vi "4461 - Create IO Channels Parallel Uneven.vi"(0 "sample mode":i32(ring)=10178 items=["Finite Samples"=10178, "Continuous Samples"=10123], 1 "Channels: Lockin":T1={"REF f (Hz)"=[0.4, 0.4], "REF phi (deg)"=[0.0, 0.0]} {"REF phi (deg)" format="%#_3g"}, 6 "error in":errorcluster, 7 "AI Buffer Size (S)":i32=10, 8 "sampling info":cluster{"Fs":dbl, "#s":dbl}, 9 "AO":T2={"AO amp (V)"=[0.1, 0.09, 0.08, 0.07, 0.06, 0.05, 0.04, 0.03], "AO DC (V)"=[0.0, 0.0, 0.0, 0.0, 0.0, 0.0, 0.0, 0.0], "AO f (Hz)"=[13.0, 13.0, 13.0, 13.0, 13.0, 13.0, 13.0, 13.0], "AO phi (deg)"=[0.0, 0.0, 0.0, 0.0, 0.0, 0.0, 0.0, 0.0], "function"=[enum."Sine Wave", enum."Sine Wave", enum."Sine Wave", enum."Sine Wave", enum."Sine Wave", enum."Sine Wave", enum."Sine Wave", enum."Sine Wave"]} {"AO DC (V)" format="%#_6p"; "AO amp (V)" format="%#_6p"}, 10 "AO Configuration":T3(array[cluster]), 11 "AI Configuration":T4(array[cluster])) -> (2 "AO Task":refnum<k21>[](array[refnum]), 3 "AI task":refnum<k21>[](array[refnum]), 4 "error out":errorcluster, 5 "phase log":dbl[](array[numeric])=[0.99999999999938, 0.99999999999938])   [LabVIEW 2016]
uses:
  <vilib>/DAQmx/write.llb/DAQmx Write (Analog 1D Wfm NChan NSamp).vi
  <vilib>/DAQmx/read.llb/DAQmx Read (Analog 1D Wfm NChan NSamp).vi
  <vilib>/DAQmx/create/channels.llb/DAQmx Create Channel (AI-Voltage-Basic).vi
  <vilib>/DAQmx/configure/timing.llb/DAQmx Timing (Sample Clock).vi
  <vilib>/DAQmx/create/channels.llb/DAQmx Create Channel (AO-Voltage-Basic).vi
  <vilib>/DAQmx/configure/trigger.llb/DAQmx Start Trigger (Digital Edge).vi
  <vilib>/DAQmx/miscellaneous.llb/DAQmx Fill In Error Info.vi
  <resource>/objmgr/daqmx.rc
panel:
  in  "AI.FilterDelay":dbl
  in  "AI.Gain":dbl
  in  "input terminal configuration":i32(ring)=-1 items=["default"=-1, "RSE"=10083, "NRSE"=10078, "Differential"=10106, "Pseudodifferential"=12529]
  in  "output terminal configuration":i32(ring)=-1 items=["Default"=-1, "RSE"=10083, "Differential"=10106, "Pseudodifferential"=12529]
  in  "SampClk.Timebase.Rate":dbl
  in  "SampQuant.SampPerChan":dbl
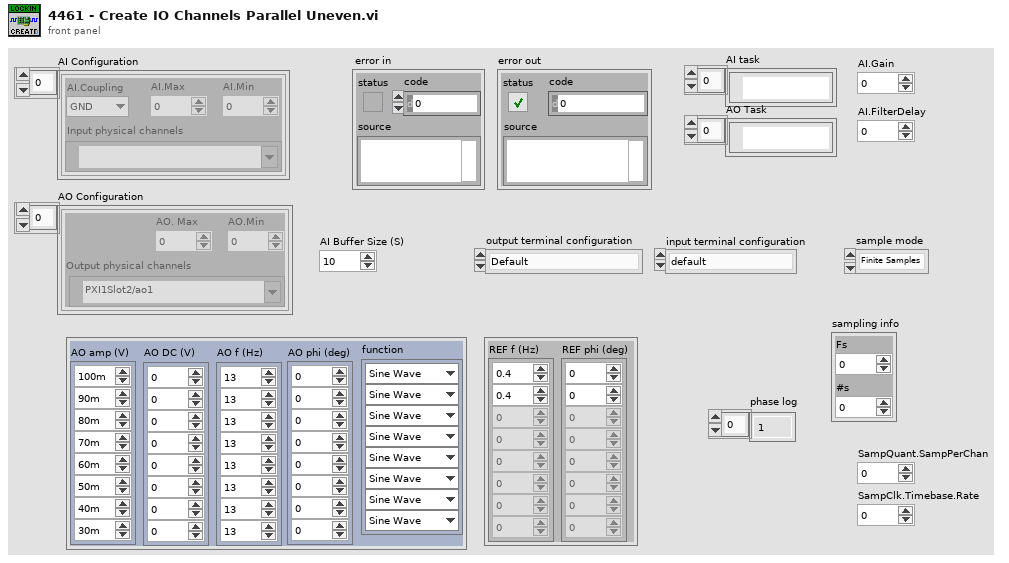
[diagram p1: front panel]
types:
  T1 = cluster{"REF f (Hz)":dbl[], "REF phi (deg)":dbl[]}
  T2 = cluster{"AO amp (V)":dbl[], "AO DC (V)":dbl[], "AO f (Hz)":dbl[], "AO phi (deg)":dbl[], "function":enum16{"Sine Wave", "Triangle Wave", "Square Wave", "Sawtooth Wave"}[]}
  T3 = cluster{"Output physical channels":tag, "AO. Max":dbl, "AO.Min":dbl}[]
  T4 = cluster{"AI.Coupling":enum16{"AC", "DC", "GND"}, "AI.Max":dbl, "AI.Min":dbl, "Input physical channels":tag}[]
  T5 = cluster{"Output physical channels":tag, "AO. Max":dbl, "AO.Min":dbl}
  T6 = cluster{"AI.Coupling":enum16{"AC", "DC", "GND"}, "AI.Max":dbl, "AI.Min":dbl, "Input physical channels":tag}
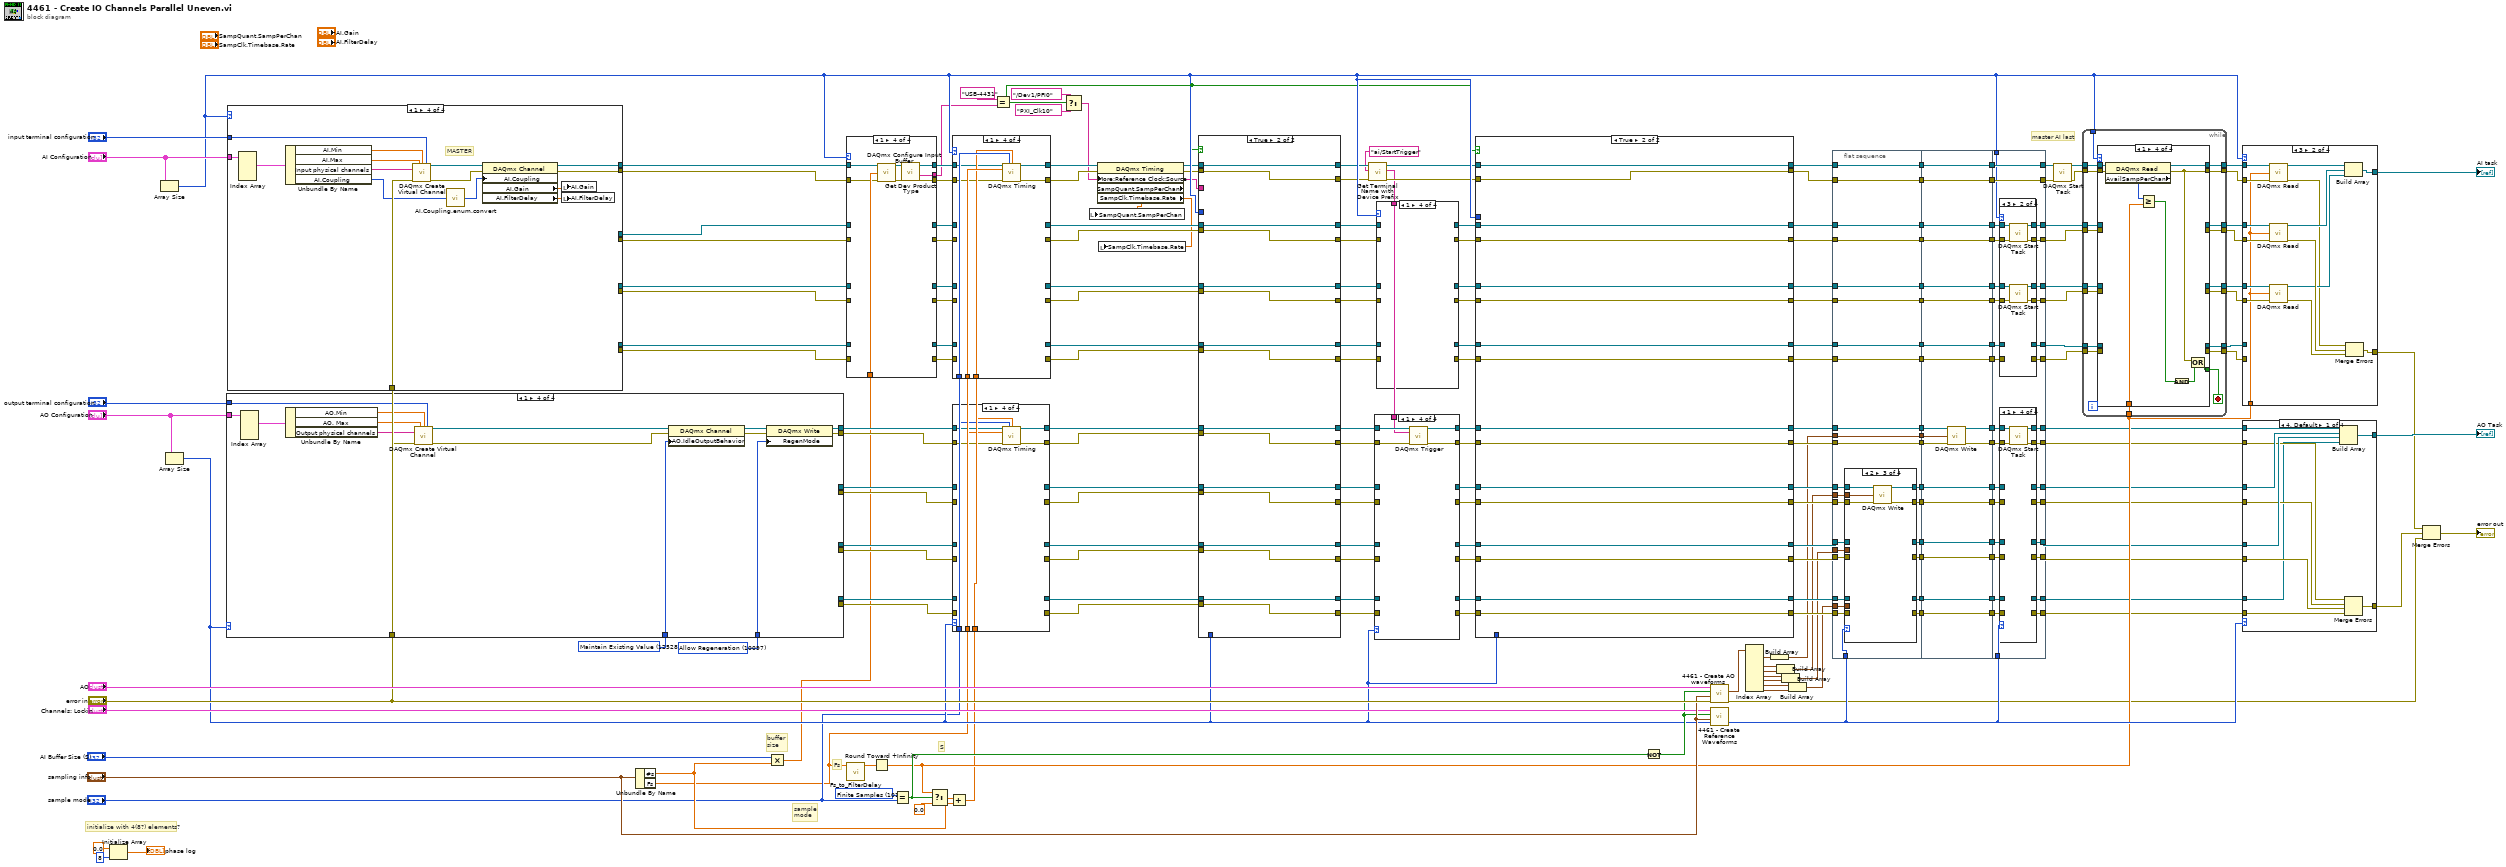
[diagram p0: block diagram]
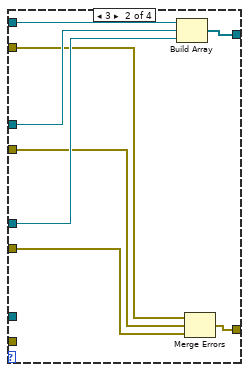
[diagram p2: hidden frame]
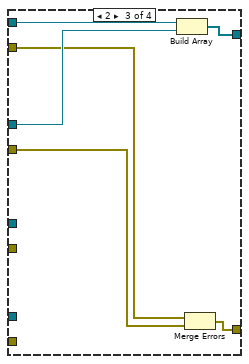
[diagram p3: hidden frame]
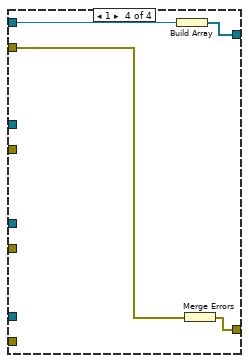
[diagram p4: hidden frame]
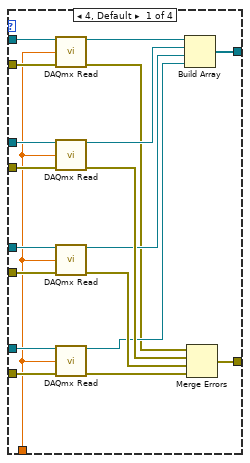
[diagram p5: hidden frame]
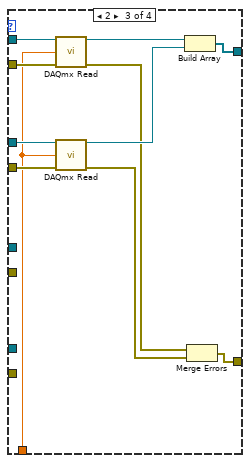
[diagram p6: hidden frame]
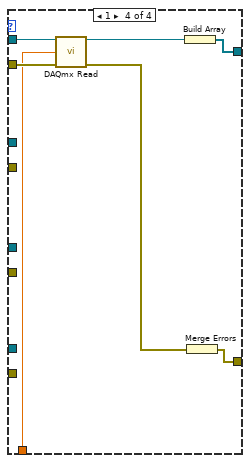
[diagram p7: hidden frame]
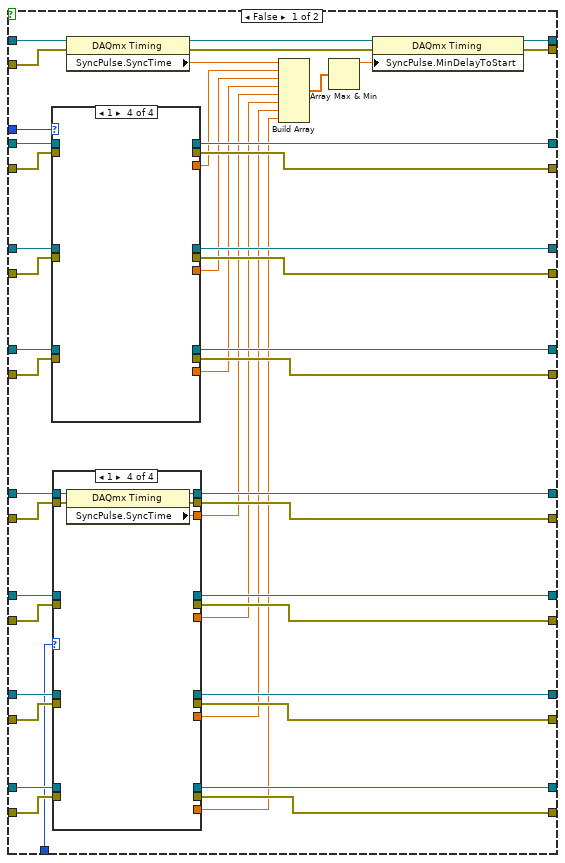
[diagram p8: hidden frame]
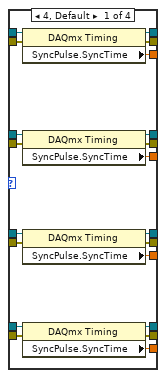
[diagram p9: hidden frame]
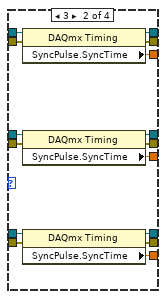
[diagram p10: hidden frame]
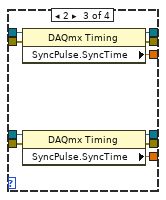
[diagram p11: hidden frame]
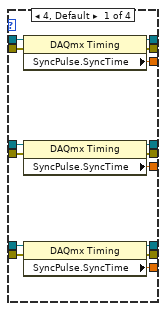
[diagram p12: hidden frame]
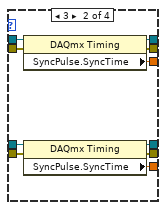
[diagram p13: hidden frame]
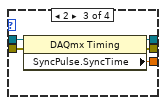
[diagram p14: hidden frame]
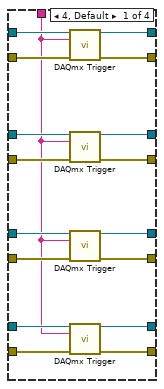
[diagram p15: hidden frame]
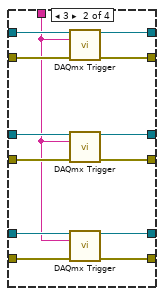
[diagram p16: hidden frame]
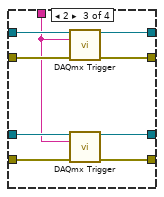
[diagram p17: hidden frame]
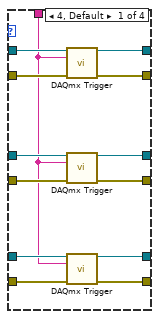
[diagram p18: hidden frame]
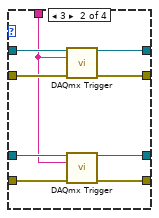
[diagram p19: hidden frame]
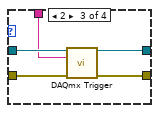
[diagram p20: hidden frame]
diagram:
  w186 = 10097 items=["Allow Regeneration"=10097, "Do Not Allow Regeneration"=10158] ("RegenMode")
  w188 = 12528 items=["Zero Volts"=12526, "High-Impedance"=12527, "Maintain Existing Value"=12528] ("AO.IdleOutputBehavior")
  w191 = 10178 items=["Finite Samples"=10178, "Continuous Samples"=10123] ("sample mode 2")
  # "master AI last"
  # "S"
  # "Fs"
  # "sample\nmode"
  # "buffer\nsize"
  # "initialize with 4(8?) elements?"
  n1 = Initialize Array(0.0 ("element"), 8 ("dimension size")) -> (→"phase log":dbl[])
  n2 = Array Size(array="AI Configuration") -> (size(s)=w179:i32)
  n3 = Array Size(array="AO Configuration") -> (size(s)=w181:i32)
  n4 = case shown="1" w181 {
    tunnel: "AO Configuration" -> [w250 w285 w310 w325]
    tunnel: "error in" -> [w242 w278 w304 w320]
    tunnel: "output terminal configuration" -> [w241 w277 w303 w319]
    tunnel: [w236 w272 w298 w314] -> w79
    tunnel: [w235 _ _ _] -> w78
    tunnel: [w234 w271 w297 _] -> w77
    tunnel: [w233 w270 _ _] -> w76
    tunnel: w188 -> [w232 w269 w296 w313]
    tunnel: [w231 w268 w295 w312] -> w58
    tunnel: [w230 w267 w294 _] -> w57
    tunnel: [w229 w266 _ _] -> w56
    tunnel: [w228 _ _ _] -> w55
    tunnel: w186 -> [w227 w265 w293 w311]
    frame 4, Default {
      n5 = Index Array(array=w250) -> (element #1=w249:T5, element #2=w243:T5, element #3=w244:T5, element #4=w245:T5)  [unwired: 4 in]
      n6 = Unbundle By Name(w249) -> ("AO.Min"=w246:dbl, "AO. Max"=w247:dbl, "Output physical channels"=w248:tag)
      n7 = Unbundle By Name(w243) -> ("AO.Min"=w226:dbl, "AO. Max"=w225:dbl, "Output physical channels"=w224:tag)
      n8 = Unbundle By Name(w244) -> ("AO.Min"=w221:dbl, "AO. Max"=w222:dbl, "Output physical channels"=w223:tag)
      n9 = Unbundle By Name(w245) -> ("AO.Min"=w220:dbl, "AO. Max"=w219:dbl, "Output physical channels"=w218:tag)
      n10 = call-poly <vilib>:"DAQmx Create Virtual Channel.vi"("maximum value"=w247, "minimum value"=w246, "output terminal configuration"=w241, "physical channels"=w248, "error in"=w242) -> ("task out"=w240:refnum<k21>, "error out"=w239:errorcluster)  [unwired: 9 in]
      n11 = call-poly <vilib>:"DAQmx Create Virtual Channel.vi"("maximum value"=w225, "minimum value"=w226, "output terminal configuration"=w241, "physical channels"=w224, "error in"=w242) -> ("task out"=w212:refnum<k21>, "error out"=w213:errorcluster)  [unwired: 9 in]
      n12 = call-poly <vilib>:"DAQmx Create Virtual Channel.vi"("maximum value"=w222, "minimum value"=w221, "output terminal configuration"=w241, "physical channels"=w223, "error in"=w242) -> ("task out"=w214:refnum<k21>, "error out"=w215:errorcluster)  [unwired: 9 in]
      n13 = call-poly <vilib>:"DAQmx Create Virtual Channel.vi"("maximum value"=w219, "minimum value"=w220, "output terminal configuration"=w241, "physical channels"=w218, "error in"=w242) -> ("task out"=w217:refnum<k21>, "error out"=w216:errorcluster)  [unwired: 9 in]
      n14 = property class="DAQmx Channel"(reference=w240, error in=w239, "AO.IdleOutputBehavior"=w232) -> (reference out=w238:refnum<k21>, error out=w237:errorcluster)
      n15 = property class="DAQmx Channel"(reference=w212, error in=w213, "AO.IdleOutputBehavior"=w232) -> (reference out=w206:refnum<k21>, error out=w207:errorcluster)
      n16 = property class="DAQmx Channel"(reference=w214, error in=w215, "AO.IdleOutputBehavior"=w232) -> (reference out=w208:refnum<k21>, error out=w209:errorcluster)
      n17 = property class="DAQmx Channel"(reference=w217, error in=w216, "AO.IdleOutputBehavior"=w232) -> (reference out=w211:refnum<k21>, error out=w210:errorcluster)
      n18 = property class="DAQmx Write"(reference=w238, error in=w237, "RegenMode"=w227) -> (reference out=w236:refnum<k21>, error out=w231:errorcluster)
      n19 = property class="DAQmx Write"(reference=w206, error in=w207, "RegenMode"=w227) -> (reference out=w234:refnum<k21>, error out=w230:errorcluster)
      n20 = property class="DAQmx Write"(reference=w208, error in=w209, "RegenMode"=w227) -> (reference out=w233:refnum<k21>, error out=w229:errorcluster)
      n21 = property class="DAQmx Write"(reference=w211, error in=w210, "RegenMode"=w227) -> (reference out=w235:refnum<k21>, error out=w228:errorcluster)
    }
    frame 3 {
      n22 = Index Array(array=w285) -> (element #1=w284:T5, element #2=w279:T5, element #3=w280:T5)  [unwired: 4 in, 1 out]
      n23 = Unbundle By Name(w284) -> ("AO.Min"=w281:dbl, "AO. Max"=w282:dbl, "Output physical channels"=w283:tag)
      n24 = Unbundle By Name(w279) -> ("AO.Min"=w264:dbl, "AO. Max"=w263:dbl, "Output physical channels"=w262:tag)
      n25 = Unbundle By Name(w280) -> ("AO.Min"=w259:dbl, "AO. Max"=w260:dbl, "Output physical channels"=w261:tag)
      n26 = call-poly <vilib>:"DAQmx Create Virtual Channel.vi"("maximum value"=w282, "minimum value"=w281, "output terminal configuration"=w277, "physical channels"=w283, "error in"=w278) -> ("task out"=w276:refnum<k21>, "error out"=w275:errorcluster)  [unwired: 9 in]
      n27 = call-poly <vilib>:"DAQmx Create Virtual Channel.vi"("maximum value"=w263, "minimum value"=w264, "output terminal configuration"=w277, "physical channels"=w262, "error in"=w278) -> ("task out"=w255:refnum<k21>, "error out"=w256:errorcluster)  [unwired: 9 in]
      n28 = call-poly <vilib>:"DAQmx Create Virtual Channel.vi"("maximum value"=w260, "minimum value"=w259, "output terminal configuration"=w277, "physical channels"=w261, "error in"=w278) -> ("task out"=w257:refnum<k21>, "error out"=w258:errorcluster)  [unwired: 9 in]
      n29 = property class="DAQmx Channel"(reference=w276, error in=w275, "AO.IdleOutputBehavior"=w269) -> (reference out=w274:refnum<k21>, error out=w273:errorcluster)
      n30 = property class="DAQmx Channel"(reference=w255, error in=w256, "AO.IdleOutputBehavior"=w269) -> (reference out=w251:refnum<k21>, error out=w252:errorcluster)
      n31 = property class="DAQmx Channel"(reference=w257, error in=w258, "AO.IdleOutputBehavior"=w269) -> (reference out=w253:refnum<k21>, error out=w254:errorcluster)
      n32 = property class="DAQmx Write"(reference=w274, error in=w273, "RegenMode"=w265) -> (reference out=w272:refnum<k21>, error out=w268:errorcluster)
      n33 = property class="DAQmx Write"(reference=w251, error in=w252, "RegenMode"=w265) -> (reference out=w271:refnum<k21>, error out=w267:errorcluster)
      n34 = property class="DAQmx Write"(reference=w253, error in=w254, "RegenMode"=w265) -> (reference out=w270:refnum<k21>, error out=w266:errorcluster)
    }
    frame 2 {
      n35 = Index Array(array=w310) -> (element #1=w309:T5, element #2=w305:T5)  [unwired: 4 in, 2 out]
      n36 = Unbundle By Name(w309) -> ("AO.Min"=w306:dbl, "AO. Max"=w307:dbl, "Output physical channels"=w308:tag)
      n37 = Unbundle By Name(w305) -> ("AO.Min"=w292:dbl, "AO. Max"=w291:dbl, "Output physical channels"=w290:tag)
      n38 = call-poly <vilib>:"DAQmx Create Virtual Channel.vi"("maximum value"=w307, "minimum value"=w306, "output terminal configuration"=w303, "physical channels"=w308, "error in"=w304) -> ("task out"=w302:refnum<k21>, "error out"=w301:errorcluster)  [unwired: 9 in]
      n39 = call-poly <vilib>:"DAQmx Create Virtual Channel.vi"("maximum value"=w291, "minimum value"=w292, "output terminal configuration"=w303, "physical channels"=w290, "error in"=w304) -> ("task out"=w288:refnum<k21>, "error out"=w289:errorcluster)  [unwired: 9 in]
      n40 = property class="DAQmx Channel"(reference=w302, error in=w301, "AO.IdleOutputBehavior"=w296) -> (reference out=w300:refnum<k21>, error out=w299:errorcluster)
      n41 = property class="DAQmx Channel"(reference=w288, error in=w289, "AO.IdleOutputBehavior"=w296) -> (reference out=w286:refnum<k21>, error out=w287:errorcluster)
      n42 = property class="DAQmx Write"(reference=w300, error in=w299, "RegenMode"=w293) -> (reference out=w298:refnum<k21>, error out=w295:errorcluster)
      n43 = property class="DAQmx Write"(reference=w286, error in=w287, "RegenMode"=w293) -> (reference out=w297:refnum<k21>, error out=w294:errorcluster)
    }
    frame 1 {
      n44 = Index Array(array=w325) -> (element #1=w324:T5)  [unwired: 4 in, 3 out]
      n45 = Unbundle By Name(w324) -> ("AO.Min"=w321:dbl, "AO. Max"=w322:dbl, "Output physical channels"=w323:tag)
      n46 = call-poly <vilib>:"DAQmx Create Virtual Channel.vi"("maximum value"=w322, "minimum value"=w321, "output terminal configuration"=w319, "physical channels"=w323, "error in"=w320) -> ("task out"=w318:refnum<k21>, "error out"=w317:errorcluster)  [unwired: 9 in]
      n47 = property class="DAQmx Channel"(reference=w318, error in=w317, "AO.IdleOutputBehavior"=w313) -> (reference out=w316:refnum<k21>, error out=w315:errorcluster)
      n48 = property class="DAQmx Write"(reference=w316, error in=w315, "RegenMode"=w311) -> (reference out=w314:refnum<k21>, error out=w312:errorcluster)
    }
  }
  n49 = case shown="1" w179 {
    tunnel: "AI Configuration" -> [w370 w405 w430 w445]
    tunnel: "error in" -> [w369 w404 w429 w444]
    tunnel: "input terminal configuration" -> [w368 w403 w428 w443]
    tunnel: [w367 w402 w427 _] -> w70
    tunnel: [w366 w401 _ _] -> w69
    tunnel: [w365 _ _ _] -> w68
    tunnel: [w364 w400 w426 _] -> w61
    tunnel: [w363 w399 _ _] -> w60
    tunnel: [w362 _ _ _] -> w59
    tunnel: [w361 w398 w425 w442] -> w32
    tunnel: [w360 w397 w424 w441] -> w31
    frame 4, Default {
      # "MASTER"
      n50 = Index Array(array=w370) -> (element #1=w359:T6, element #2=w353:T6, element #3=w352:T6, element #4=w351:T6)  [unwired: 4 in]
      n51 = Unbundle By Name(w359) -> ("AI.Min"=w354:dbl, "AI.Max"=w355:dbl, "Input physical channels"=w358:tag, "AI.Coupling"=w348:enum16{"AC", "DC", "GND"})
      n52 = Unbundle By Name(w353) -> ("AI.Min"=w347:dbl, "AI.Max"=w346:dbl, "Input physical channels"=w343:tag, "AI.Coupling"=w330:enum16{"AC", "DC", "GND"})
      n53 = Unbundle By Name(w352) -> ("AI.Min"=w338:dbl, "AI.Max"=w339:dbl, "Input physical channels"=w342:tag, "AI.Coupling"=w331:enum16{"AC", "DC", "GND"})
      n54 = Unbundle By Name(w351) -> ("AI.Min"=w337:dbl, "AI.Max"=w336:dbl, "Input physical channels"=w333:tag, "AI.Coupling"=w332:enum16{"AC", "DC", "GND"})
      n55 = call-poly <vilib>:"DAQmx Create Virtual Channel.vi"("maximum value"=w355, "minimum value"=w354, "input terminal configuration"=w368, "physical channels"=w358, "error in"=w369) -> ("task out"=w357:refnum<k21>, "error out"=w356:errorcluster)  [unwired: 9 in]
      n56 = call-poly <vilib>:"DAQmx Create Virtual Channel.vi"("maximum value"=w346, "minimum value"=w347, "input terminal configuration"=w368, "physical channels"=w343, "error in"=w369) -> ("task out"=w344:refnum<k21>, "error out"=w345:errorcluster)  [unwired: 9 in]
      n57 = call-poly <vilib>:"DAQmx Create Virtual Channel.vi"("maximum value"=w339, "minimum value"=w338, "input terminal configuration"=w368, "physical channels"=w342, "error in"=w369) -> ("task out"=w341:refnum<k21>, "error out"=w340:errorcluster)  [unwired: 9 in]
      n58 = call-poly <vilib>:"DAQmx Create Virtual Channel.vi"("maximum value"=w336, "minimum value"=w337, "input terminal configuration"=w368, "physical channels"=w333, "error in"=w369) -> ("task out"=w334:refnum<k21>, "error out"=w335:errorcluster)  [unwired: 9 in]
      n59 = call "AI.Coupling.enum.convert.vi"("AI.Coupling"=w348) -> ("Numeric"=w329:i32)
      n60 = call "AI.Coupling.enum.convert.vi"("AI.Coupling"=w331) -> ("Numeric"=w327:i32)
      n61 = call "AI.Coupling.enum.convert.vi"("AI.Coupling"=w330) -> ("Numeric"=w328:i32)
      n62 = call "AI.Coupling.enum.convert.vi"("AI.Coupling"=w332) -> ("Numeric"=w326:i32)
      n63 = property class="DAQmx Channel"(reference=w357, error in=w356, "AI.Coupling"=w329) -> (reference out=w361:refnum<k21>, error out=w360:errorcluster, "AI.Gain"=w350:dbl, "AI.FilterDelay"=w349:dbl)
      n64 = property class="DAQmx Channel"(reference=w344, error in=w345, "AI.Coupling"=w328) -> (reference out=w367:refnum<k21>, error out=w364:errorcluster)
      n65 = property class="DAQmx Channel"(reference=w341, error in=w340, "AI.Coupling"=w327) -> (reference out=w366:refnum<k21>, error out=w363:errorcluster)
      n66 = property class="DAQmx Channel"(reference=w334, error in=w335, "AI.Coupling"=w326) -> (reference out=w365:refnum<k21>, error out=w362:errorcluster)
      n67 = local write "AI.Gain"(w350) -> ()
      n68 = local write "AI.FilterDelay"(w349) -> ()
    }
    frame 3 {
      # "MASTER"
      n69 = Index Array(array=w405) -> (element #1=w396:T6, element #2=w390:T6, element #3=w389:T6)  [unwired: 4 in, 1 out]
      n70 = Unbundle By Name(w396) -> ("AI.Min"=w391:dbl, "AI.Max"=w392:dbl, "Input physical channels"=w395:tag, "AI.Coupling"=w386:enum16{"AC", "DC", "GND"})
      n71 = Unbundle By Name(w390) -> ("AI.Min"=w385:dbl, "AI.Max"=w384:dbl, "Input physical channels"=w381:tag, "AI.Coupling"=w374:enum16{"AC", "DC", "GND"})
      n72 = Unbundle By Name(w389) -> ("AI.Min"=w376:dbl, "AI.Max"=w377:dbl, "Input physical channels"=w380:tag, "AI.Coupling"=w375:enum16{"AC", "DC", "GND"})
      n73 = call-poly <vilib>:"DAQmx Create Virtual Channel.vi"("maximum value"=w392, "minimum value"=w391, "input terminal configuration"=w403, "physical channels"=w395, "error in"=w404) -> ("task out"=w394:refnum<k21>, "error out"=w393:errorcluster)  [unwired: 9 in]
      n74 = call-poly <vilib>:"DAQmx Create Virtual Channel.vi"("maximum value"=w384, "minimum value"=w385, "input terminal configuration"=w403, "physical channels"=w381, "error in"=w404) -> ("task out"=w382:refnum<k21>, "error out"=w383:errorcluster)  [unwired: 9 in]
      n75 = call-poly <vilib>:"DAQmx Create Virtual Channel.vi"("maximum value"=w377, "minimum value"=w376, "input terminal configuration"=w403, "physical channels"=w380, "error in"=w404) -> ("task out"=w379:refnum<k21>, "error out"=w378:errorcluster)  [unwired: 9 in]
      n76 = call "AI.Coupling.enum.convert.vi"("AI.Coupling"=w386) -> ("Numeric"=w373:i32)
      n77 = call "AI.Coupling.enum.convert.vi"("AI.Coupling"=w375) -> ("Numeric"=w371:i32)
      n78 = call "AI.Coupling.enum.convert.vi"("AI.Coupling"=w374) -> ("Numeric"=w372:i32)
      n79 = property class="DAQmx Channel"(reference=w394, error in=w393, "AI.Coupling"=w373) -> (reference out=w398:refnum<k21>, error out=w397:errorcluster, "AI.Gain"=w388:dbl, "AI.FilterDelay"=w387:dbl)
      n80 = property class="DAQmx Channel"(reference=w382, error in=w383, "AI.Coupling"=w372) -> (reference out=w402:refnum<k21>, error out=w400:errorcluster)
      n81 = property class="DAQmx Channel"(reference=w379, error in=w378, "AI.Coupling"=w371) -> (reference out=w401:refnum<k21>, error out=w399:errorcluster)
      n82 = local write "AI.Gain"(w388) -> ()
      n83 = local write "AI.FilterDelay"(w387) -> ()
    }
    frame 2 {
      # "MASTER"
      n84 = Index Array(array=w430) -> (element #1=w423:T6, element #2=w417:T6)  [unwired: 4 in, 2 out]
      n85 = Unbundle By Name(w423) -> ("AI.Min"=w418:dbl, "AI.Max"=w419:dbl, "Input physical channels"=w422:tag, "AI.Coupling"=w414:enum16{"AC", "DC", "GND"})
      n86 = Unbundle By Name(w417) -> ("AI.Min"=w413:dbl, "AI.Max"=w412:dbl, "Input physical channels"=w409:tag, "AI.Coupling"=w408:enum16{"AC", "DC", "GND"})
      n87 = call-poly <vilib>:"DAQmx Create Virtual Channel.vi"("maximum value"=w419, "minimum value"=w418, "input terminal configuration"=w428, "physical channels"=w422, "error in"=w429) -> ("task out"=w421:refnum<k21>, "error out"=w420:errorcluster)  [unwired: 9 in]
      n88 = call-poly <vilib>:"DAQmx Create Virtual Channel.vi"("maximum value"=w412, "minimum value"=w413, "input terminal configuration"=w428, "physical channels"=w409, "error in"=w429) -> ("task out"=w410:refnum<k21>, "error out"=w411:errorcluster)  [unwired: 9 in]
      n89 = call "AI.Coupling.enum.convert.vi"("AI.Coupling"=w414) -> ("Numeric"=w407:i32)
      n90 = call "AI.Coupling.enum.convert.vi"("AI.Coupling"=w408) -> ("Numeric"=w406:i32)
      n91 = property class="DAQmx Channel"(reference=w421, error in=w420, "AI.Coupling"=w407) -> (reference out=w425:refnum<k21>, error out=w424:errorcluster, "AI.Gain"=w416:dbl, "AI.FilterDelay"=w415:dbl)
      n92 = property class="DAQmx Channel"(reference=w410, error in=w411, "AI.Coupling"=w406) -> (reference out=w427:refnum<k21>, error out=w426:errorcluster)
      n93 = local write "AI.Gain"(w416) -> ()
      n94 = local write "AI.FilterDelay"(w415) -> ()
    }
    frame 1 {
      # "MASTER"
      n95 = Index Array(array=w445) -> (element #1=w440:T6)  [unwired: 4 in, 3 out]
      n96 = Unbundle By Name(w440) -> ("AI.Min"=w435:dbl, "AI.Max"=w436:dbl, "Input physical channels"=w439:tag, "AI.Coupling"=w432:enum16{"AC", "DC", "GND"})
      n97 = call-poly <vilib>:"DAQmx Create Virtual Channel.vi"("maximum value"=w436, "minimum value"=w435, "input terminal configuration"=w443, "physical channels"=w439, "error in"=w444) -> ("task out"=w438:refnum<k21>, "error out"=w437:errorcluster)  [unwired: 9 in]
      n98 = call "AI.Coupling.enum.convert.vi"("AI.Coupling"=w432) -> ("Numeric"=w431:i32)
      n99 = property class="DAQmx Channel"(reference=w438, error in=w437, "AI.Coupling"=w431) -> (reference out=w442:refnum<k21>, error out=w441:errorcluster, "AI.Gain"=w434:dbl, "AI.FilterDelay"=w433:dbl)
      n100 = local write "AI.Gain"(w434) -> ()
      n101 = local write "AI.FilterDelay"(w433) -> ()
    }
  }
  n102 = Unbundle By Name("sampling info") -> ("#s"=w187:dbl, "Fs"=w3:dbl)
  n103 = Multiply(x="AI Buffer Size (S)", y=w187) -> (x*y=w1:dbl)
  n104 = case shown="1" w179 {
    tunnel: w70 -> [w465 w481 w493 _]
    tunnel: w69 -> [w464 w480 _ _]
    tunnel: w68 -> [w463 _ _ _]
    tunnel: [w462 _ _ _] -> w67
    tunnel: [w461 w479 _ _] -> w66
    tunnel: [w460 w478 _ _] -> w65
    tunnel: [w459 _ _ _] -> w64
    tunnel: [w458 w477 w492 _] -> w63
    tunnel: [w457 w476 w491 _] -> w62
    tunnel: w61 -> [w456 w475 w490 _]
    tunnel: w60 -> [w455 w474 _ _]
    tunnel: w59 -> [w454 _ _ _]
    tunnel: w1 -> [w453 w473 w489 w501]
    tunnel: w32 -> [w452 w472 w488 w500]
    tunnel: w31 -> [w451 w471 w487 w499]
    tunnel: [w448 w468 w484 w496] -> w14
    tunnel: [w447 w467 w483 w495] -> w13
    tunnel: [w446 w466 w482 w494] -> w11
    frame 4, Default {
      n105 = call <vilib>:"DAQmx Configure Input Buffer.vi"("task/channels in"=w452, "buffer size (in samples per channel)"=w453, "error in"=w451) -> ("task out"=w450:refnum<k21>, "error out"=w449:errorcluster)  [unwired: 11 in]
      n106 = call <vilib>:"DAQmx Configure Input Buffer.vi"("task/channels in"=w465, "buffer size (in samples per channel)"=w453, "error in"=w456) -> ("task out"=w457:refnum<k21>, "error out"=w458:errorcluster)  [unwired: 11 in]
      n107 = call <vilib>:"DAQmx Configure Input Buffer.vi"("task/channels in"=w464, "buffer size (in samples per channel)"=w453, "error in"=w455) -> ("task out"=w461:refnum<k21>, "error out"=w460:errorcluster)  [unwired: 11 in]
      n108 = call <vilib>:"DAQmx Configure Input Buffer.vi"("task/channels in"=w463, "buffer size (in samples per channel)"=w453, "error in"=w454) -> ("task out"=w462:refnum<k21>, "error out"=w459:errorcluster)  [unwired: 11 in]
      n109 = call "Get Dev Product Type.vi"("error in (no error)"=w449, "Refnum in"=w450) -> ("error out"=w448:errorcluster, "ProductType"=w446:string, "Refnum out"=w447:refnum<k21>)  [unwired: 7 in]
    }
    frame 3 {
      n110 = call <vilib>:"DAQmx Configure Input Buffer.vi"("task/channels in"=w472, "buffer size (in samples per channel)"=w473, "error in"=w471) -> ("task out"=w470:refnum<k21>, "error out"=w469:errorcluster)  [unwired: 11 in]
      n111 = call <vilib>:"DAQmx Configure Input Buffer.vi"("task/channels in"=w481, "buffer size (in samples per channel)"=w473, "error in"=w475) -> ("task out"=w476:refnum<k21>, "error out"=w477:errorcluster)  [unwired: 11 in]
      n112 = call <vilib>:"DAQmx Configure Input Buffer.vi"("task/channels in"=w480, "buffer size (in samples per channel)"=w473, "error in"=w474) -> ("task out"=w479:refnum<k21>, "error out"=w478:errorcluster)  [unwired: 11 in]
      n113 = call "Get Dev Product Type.vi"("error in (no error)"=w469, "Refnum in"=w470) -> ("error out"=w468:errorcluster, "ProductType"=w466:string, "Refnum out"=w467:refnum<k21>)  [unwired: 7 in]
    }
    frame 2 {
      n114 = call <vilib>:"DAQmx Configure Input Buffer.vi"("task/channels in"=w488, "buffer size (in samples per channel)"=w489, "error in"=w487) -> ("task out"=w486:refnum<k21>, "error out"=w485:errorcluster)  [unwired: 11 in]
      n115 = call <vilib>:"DAQmx Configure Input Buffer.vi"("task/channels in"=w493, "buffer size (in samples per channel)"=w489, "error in"=w490) -> ("task out"=w491:refnum<k21>, "error out"=w492:errorcluster)  [unwired: 11 in]
      n116 = call "Get Dev Product Type.vi"("error in (no error)"=w485, "Refnum in"=w486) -> ("error out"=w484:errorcluster, "ProductType"=w482:string, "Refnum out"=w483:refnum<k21>)  [unwired: 7 in]
    }
    frame 1 {
      n117 = call <vilib>:"DAQmx Configure Input Buffer.vi"("task/channels in"=w500, "buffer size (in samples per channel)"=w501, "error in"=w499) -> ("task out"=w498:refnum<k21>, "error out"=w497:errorcluster)  [unwired: 11 in]
      n118 = call "Get Dev Product Type.vi"("error in (no error)"=w497, "Refnum in"=w498) -> ("error out"=w496:errorcluster, "ProductType"=w494:string, "Refnum out"=w495:refnum<k21>)  [unwired: 7 in]
    }
  }
  n119 = call "Fs_to_FilterDelay.vi"("Fs"=w3) -> ("Total Filter Delay (samples)"=w194:dbl)  [unwired: 10 in]
  n120 = Round Toward +Infinity(x=w194) -> (ceil(x): smallest int >= x=w180:dbl)
  n121 = Equal?(x=w191, y="sample mode") -> (x = y?=w184:bool)
  n122 = Select(t=w180, s=w184, f=0.0) -> (s? t:f=w192:dbl)
  n123 = Add(x=w192, y=w187) -> (x+y=w2:dbl)
  n124 = case shown="1" w179 {
    tunnel: [w520 w535 w546 w553] -> w145
    tunnel: [w519 w534 w545 w552] -> w136
    tunnel: [w518 w533 w544 _] -> w135
    tunnel: [w517 w532 w543 _] -> w134
    tunnel: [w516 w531 _ _] -> w129
    tunnel: [w515 w530 _ _] -> w128
    tunnel: [w514 _ _ _] -> w127
    tunnel: [w513 _ _ _] -> w126
    tunnel: w67 -> [w512 _ _ _]
    tunnel: w66 -> [w511 w529 _ _]
    tunnel: w65 -> [w510 w528 _ _]
    tunnel: w64 -> [w509 _ _ _]
    tunnel: w63 -> [w508 w527 w542 _]
    tunnel: w62 -> [w507 w526 w541 _]
    tunnel: "sample mode" -> [w506 w525 w540 w551]
    tunnel: w3 -> [w505 w524 w539 w550]
    tunnel: w2 -> [w504 w523 w538 w549]
    tunnel: w14 -> [w503 w522 w537 w548]
    tunnel: w13 -> [w502 w521 w536 w547]
    frame 4, Default {
      n125 = call-poly <vilib>:"DAQmx Timing.vi"("task/channels in"=w502, "sample mode"=w506, "samples per channel"=w504, "rate"=w505, "error in"=w503) -> ("task out"=w520:refnum<k21>, "error out"=w519:errorcluster)  [unwired: 9 in]
      n126 = call-poly <vilib>:"DAQmx Timing.vi"("task/channels in"=w507, "sample mode"=w506, "samples per channel"=w504, "rate"=w505, "error in"=w508) -> ("task out"=w518:refnum<k21>, "error out"=w517:errorcluster)  [unwired: 9 in]
      n127 = call-poly <vilib>:"DAQmx Timing.vi"("task/channels in"=w511, "sample mode"=w506, "samples per channel"=w504, "rate"=w505, "error in"=w510) -> ("task out"=w515:refnum<k21>, "error out"=w516:errorcluster)  [unwired: 9 in]
      n128 = call-poly <vilib>:"DAQmx Timing.vi"("task/channels in"=w512, "sample mode"=w506, "samples per channel"=w504, "rate"=w505, "error in"=w509) -> ("task out"=w514:refnum<k21>, "error out"=w513:errorcluster)  [unwired: 9 in]
    }
    frame 3 {
      n129 = call-poly <vilib>:"DAQmx Timing.vi"("task/channels in"=w521, "sample mode"=w525, "samples per channel"=w523, "rate"=w524, "error in"=w522) -> ("task out"=w535:refnum<k21>, "error out"=w534:errorcluster)  [unwired: 9 in]
      n130 = call-poly <vilib>:"DAQmx Timing.vi"("task/channels in"=w526, "sample mode"=w525, "samples per channel"=w523, "rate"=w524, "error in"=w527) -> ("task out"=w533:refnum<k21>, "error out"=w532:errorcluster)  [unwired: 9 in]
      n131 = call-poly <vilib>:"DAQmx Timing.vi"("task/channels in"=w529, "sample mode"=w525, "samples per channel"=w523, "rate"=w524, "error in"=w528) -> ("task out"=w530:refnum<k21>, "error out"=w531:errorcluster)  [unwired: 9 in]
    }
    frame 2 {
      n132 = call-poly <vilib>:"DAQmx Timing.vi"("task/channels in"=w536, "sample mode"=w540, "samples per channel"=w538, "rate"=w539, "error in"=w537) -> ("task out"=w546:refnum<k21>, "error out"=w545:errorcluster)  [unwired: 9 in]
      n133 = call-poly <vilib>:"DAQmx Timing.vi"("task/channels in"=w541, "sample mode"=w540, "samples per channel"=w538, "rate"=w539, "error in"=w542) -> ("task out"=w544:refnum<k21>, "error out"=w543:errorcluster)  [unwired: 9 in]
    }
    frame 1 {
      n134 = call-poly <vilib>:"DAQmx Timing.vi"("task/channels in"=w547, "sample mode"=w551, "samples per channel"=w549, "rate"=w550, "error in"=w548) -> ("task out"=w553:refnum<k21>, "error out"=w552:errorcluster)  [unwired: 9 in]
    }
  }
  n135 = case shown="1" w181 {
    tunnel: w79 -> [w572 w587 w598 w605]
    tunnel: w78 -> [w571 _ _ _]
    tunnel: w77 -> [w570 w586 w597 _]
    tunnel: w76 -> [w569 w585 _ _]
    tunnel: [w568 w584 w596 _] -> w75
    tunnel: [w567 _ _ _] -> w74
    tunnel: [w566 _ _ _] -> w73
    tunnel: [w565 w583 _ _] -> w72
    tunnel: [w564 w582 w595 w604] -> w71
    tunnel: "sample mode" -> [w563 w581 w594 w603]
    tunnel: w3 -> [w562 w580 w593 w602]
    tunnel: w2 -> [w554 w573 w588 w599]
    tunnel: w58 -> [w561 w579 w592 w601]
    tunnel: w57 -> [w560 w578 w591 _]
    tunnel: w56 -> [w559 w577 _ _]
    tunnel: w55 -> [w558 _ _ _]
    tunnel: [w557 w576 w590 w600] -> w8
    tunnel: [w556 w575 w589 _] -> w38
    tunnel: [w555 w574 _ _] -> w37
    frame 4, Default {
      n136 = call-poly <vilib>:"DAQmx Timing.vi"("task/channels in"=w572, "sample mode"=w563, "samples per channel"=w554, "rate"=w562, "error in"=w561) -> ("task out"=w564:refnum<k21>, "error out"=w557:errorcluster)  [unwired: 9 in]
      n137 = call-poly <vilib>:"DAQmx Timing.vi"("task/channels in"=w570, "sample mode"=w563, "samples per channel"=w554, "rate"=w562, "error in"=w560) -> ("task out"=w568:refnum<k21>, "error out"=w556:errorcluster)  [unwired: 9 in]
      n138 = call-poly <vilib>:"DAQmx Timing.vi"("task/channels in"=w569, "sample mode"=w563, "samples per channel"=w554, "rate"=w562, "error in"=w559) -> ("task out"=w565:refnum<k21>, "error out"=w555:errorcluster)  [unwired: 9 in]
      n139 = call-poly <vilib>:"DAQmx Timing.vi"("task/channels in"=w571, "sample mode"=w563, "samples per channel"=w554, "rate"=w562, "error in"=w558) -> ("task out"=w566:refnum<k21>, "error out"=w567:errorcluster)  [unwired: 9 in]
    }
    frame 3 {
      n140 = call-poly <vilib>:"DAQmx Timing.vi"("task/channels in"=w587, "sample mode"=w581, "samples per channel"=w573, "rate"=w580, "error in"=w579) -> ("task out"=w582:refnum<k21>, "error out"=w576:errorcluster)  [unwired: 9 in]
      n141 = call-poly <vilib>:"DAQmx Timing.vi"("task/channels in"=w586, "sample mode"=w581, "samples per channel"=w573, "rate"=w580, "error in"=w578) -> ("task out"=w584:refnum<k21>, "error out"=w575:errorcluster)  [unwired: 9 in]
      n142 = call-poly <vilib>:"DAQmx Timing.vi"("task/channels in"=w585, "sample mode"=w581, "samples per channel"=w573, "rate"=w580, "error in"=w577) -> ("task out"=w583:refnum<k21>, "error out"=w574:errorcluster)  [unwired: 9 in]
    }
    frame 2 {
      n143 = call-poly <vilib>:"DAQmx Timing.vi"("task/channels in"=w598, "sample mode"=w594, "samples per channel"=w588, "rate"=w593, "error in"=w592) -> ("task out"=w595:refnum<k21>, "error out"=w590:errorcluster)  [unwired: 9 in]
      n144 = call-poly <vilib>:"DAQmx Timing.vi"("task/channels in"=w597, "sample mode"=w594, "samples per channel"=w588, "rate"=w593, "error in"=w591) -> ("task out"=w596:refnum<k21>, "error out"=w589:errorcluster)  [unwired: 9 in]
    }
    frame 1 {
      n145 = call-poly <vilib>:"DAQmx Timing.vi"("task/channels in"=w605, "sample mode"=w603, "samples per channel"=w599, "rate"=w602, "error in"=w601) -> ("task out"=w604:refnum<k21>, "error out"=w600:errorcluster)  [unwired: 9 in]
    }
  }
  n146 = Equal?(x="USB-4431" ("ProductType"), y=w11) -> (x = y?=w7:bool)
  n147 = Select(t=tag "/Dev1/PFI0" ("RefClk.Src"), s=w7, f=tag "PXI_Clk10" ("RefClk.Src")) -> (s? t:f=w9:tag)
  n148 = property class="DAQmx Timing"(reference=w145, error in=w136, "More:Reference Clock:Source"=w9) -> (reference out=w95:refnum<k21>, error out=w10:errorcluster, "SampQuant.SampPerChan"=w34:dbl, "SampClk.Timebase.Rate"=w33:dbl)
  n149 = local write "SampQuant.SampPerChan"(w34) -> ()
  n150 = local write "SampClk.Timebase.Rate"(w33) -> ()
  n151 = case shown="True" w7 {
    tunnel: [w642 w736] -> w142
    tunnel: [w641 w735] -> w141
    tunnel: w135 -> [w640 w734]
    tunnel: w134 -> [w639 w733]
    tunnel: [w638 w734] -> w133
    tunnel: [w637 w733] -> w132
    tunnel: [w636 w731] -> w131
    tunnel: [w635 w732] -> w130
    tunnel: w129 -> [w634 w731]
    tunnel: w128 -> [w633 w732]
    tunnel: w127 -> [w632 w730]
    tunnel: w126 -> [w631 w729]
    tunnel: [w630 w730] -> w125
    tunnel: [w629 w729] -> w124
    tunnel: [w628 w728] -> w122
    tunnel: [w627 w727] -> w121
    tunnel: [w626 w725] -> w118
    tunnel: [w625 w726] -> w117
    tunnel: [w624 w724] -> w116
    tunnel: [w623 w723] -> w115
    tunnel: [w622 w721] -> w114
    tunnel: [w621 w722] -> w113
    tunnel: w95 -> [w620 w736]
    tunnel: w75 -> [w619 w726]
    tunnel: w74 -> [w618 w721]
    tunnel: w73 -> [w617 w722]
    tunnel: w72 -> [w616 w724]
    tunnel: w71 -> [w615 w728]
    tunnel: w38 -> [w613 w725]
    tunnel: w37 -> [w612 w723]
    tunnel: w10 -> [w609 w735]
    tunnel: w9 -> [w608 _]
    tunnel: w179 -> [w606 _]
    tunnel: w8 -> [w614 w727]
    tunnel: w181 -> [w607 _]
    frame False {
      n152 = call "Get Terminal Name with Device Prefix.vi"("error in (no error)"=w609, "Local Terminal Name"="SyncPulse", "task/channels in"=w620) -> ("error out"=w641:errorcluster, "Terminal Name with Device Prefix"=w610:tag, "task out"=w642:refnum<k21>)  [unwired: 6 in]
      n153 = case shown="1" w607 {
        tunnel: [w660 w674 w684 w690] -> w628
        tunnel: [w659 w673 w683 w689] -> w627
        tunnel: [w658 w672 w682 _] -> w626
        tunnel: [w657 w671 w681 _] -> w625
        tunnel: [w656 w670 _ _] -> w624
        tunnel: [w655 w669 _ _] -> w623
        tunnel: [w654 _ _ _] -> w622
        tunnel: [w653 _ _ _] -> w621
        tunnel: w619 -> [w652 w668 w680 _]
        tunnel: w618 -> [w651 _ _ _]
        tunnel: w617 -> [w650 _ _ _]
        tunnel: w616 -> [w649 w667 _ _]
        tunnel: w615 -> [w648 w666 w679 w688]
        tunnel: w614 -> [w647 w665 w678 w687]
        tunnel: w613 -> [w646 w664 w677 _]
        tunnel: w612 -> [w645 w663 _ _]
        tunnel: w610 -> [w644 w662 w676 w686]
        tunnel: w608 -> [w643 w661 w675 w685]
        frame 4, Default {
          n154 = property class="DAQmx Timing"(reference=w648, error in=w647, "More:Reference Clock:Source"=w643, "More:Synchronization Pulse:Source"=w644) -> (reference out=w660:refnum<k21>, error out=w659:errorcluster)
          n155 = property class="DAQmx Timing"(reference=w652, error in=w646, "More:Reference Clock:Source"=w643, "More:Synchronization Pulse:Source"=w644) -> (reference out=w657:refnum<k21>, error out=w658:errorcluster)
          n156 = property class="DAQmx Timing"(reference=w649, error in=w645, "More:Reference Clock:Source"=w643, "More:Synchronization Pulse:Source"=w644) -> (reference out=w656:refnum<k21>, error out=w655:errorcluster)
          n157 = property class="DAQmx Timing"(reference=w650, error in=w651, "More:Reference Clock:Source"=w643, "More:Synchronization Pulse:Source"=w644) -> (reference out=w653:refnum<k21>, error out=w654:errorcluster)
        }
        frame 3 {
          n158 = property class="DAQmx Timing"(reference=w666, error in=w665, "More:Reference Clock:Source"=w661, "More:Synchronization Pulse:Source"=w662) -> (reference out=w674:refnum<k21>, error out=w673:errorcluster)
          n159 = property class="DAQmx Timing"(reference=w668, error in=w664, "More:Reference Clock:Source"=w661, "More:Synchronization Pulse:Source"=w662) -> (reference out=w671:refnum<k21>, error out=w672:errorcluster)
          n160 = property class="DAQmx Timing"(reference=w667, error in=w663, "More:Reference Clock:Source"=w661, "More:Synchronization Pulse:Source"=w662) -> (reference out=w670:refnum<k21>, error out=w669:errorcluster)
        }
        frame 2 {
          n161 = property class="DAQmx Timing"(reference=w679, error in=w678, "More:Reference Clock:Source"=w675, "More:Synchronization Pulse:Source"=w676) -> (reference out=w684:refnum<k21>, error out=w683:errorcluster)
          n162 = property class="DAQmx Timing"(reference=w680, error in=w677, "More:Reference Clock:Source"=w675, "More:Synchronization Pulse:Source"=w676) -> (reference out=w681:refnum<k21>, error out=w682:errorcluster)
        }
        frame 1 {
          n163 = property class="DAQmx Timing"(reference=w688, error in=w687, "More:Reference Clock:Source"=w685, "More:Synchronization Pulse:Source"=w686) -> (reference out=w690:refnum<k21>, error out=w689:errorcluster)
        }
      }
      n164 = case shown="3" w606 {
        tunnel: w640 -> [w704 w714 w720 _]
        tunnel: w639 -> [w703 w713 w719 _]
        tunnel: [w702 w712 w718 _] -> w638
        tunnel: [w701 w711 w717 _] -> w637
        tunnel: [w700 w710 _ _] -> w636
        tunnel: [w699 w709 _ _] -> w635
        tunnel: w634 -> [w698 w708 _ _]
        tunnel: w633 -> [w697 w707 _ _]
        tunnel: w632 -> [w696 _ _ _]
        tunnel: w631 -> [w695 _ _ _]
        tunnel: [w694 _ _ _] -> w630
        tunnel: [w693 _ _ _] -> w629
        tunnel: w610 -> [w692 w706 w716 _]
        tunnel: w608 -> [w691 w705 w715 _]
        frame 4, Default {
          n165 = property class="DAQmx Timing"(reference=w704, error in=w703, "More:Reference Clock:Source"=w691, "More:Synchronization Pulse:Source"=w692) -> (reference out=w702:refnum<k21>, error out=w701:errorcluster)
          n166 = property class="DAQmx Timing"(reference=w697, error in=w698, "More:Reference Clock:Source"=w691, "More:Synchronization Pulse:Source"=w692) -> (reference out=w699:refnum<k21>, error out=w700:errorcluster)
          n167 = property class="DAQmx Timing"(reference=w696, error in=w695, "More:Reference Clock:Source"=w691, "More:Synchronization Pulse:Source"=w692) -> (reference out=w694:refnum<k21>, error out=w693:errorcluster)
        }
        frame 3 {
          n168 = property class="DAQmx Timing"(reference=w714, error in=w713, "More:Reference Clock:Source"=w705, "More:Synchronization Pulse:Source"=w706) -> (reference out=w712:refnum<k21>, error out=w711:errorcluster)
          n169 = property class="DAQmx Timing"(reference=w707, error in=w708, "More:Reference Clock:Source"=w705, "More:Synchronization Pulse:Source"=w706) -> (reference out=w709:refnum<k21>, error out=w710:errorcluster)
        }
        frame 2 {
          n170 = property class="DAQmx Timing"(reference=w720, error in=w719, "More:Reference Clock:Source"=w715, "More:Synchronization Pulse:Source"=w716) -> (reference out=w718:refnum<k21>, error out=w717:errorcluster)
        }
        frame 1 {
        }
      }
    }
    frame True {
    }
  }
  n171 = call "Get Terminal Name with Device Prefix.vi"("error in (no error)"=w141, "Local Terminal Name"="ai/StartTrigger", "task/channels in"=w142) -> ("error out"=w139:errorcluster, "Terminal Name with Device Prefix"=w112:tag, "task out"=w140:refnum<k21>)  [unwired: 6 in]
  n172 = case shown="1" w181 {
    tunnel: w122 -> [w753 w766 w775 w780]
    tunnel: w121 -> [w752 w765 w774 w779]
    tunnel: [w751 w764 w773 w778] -> w120
    tunnel: [w750 w763 w772 w777] -> w119
    tunnel: w118 -> [w749 w762 w771 _]
    tunnel: w117 -> [w748 w761 w770 _]
    tunnel: w116 -> [w747 w760 _ _]
    tunnel: w115 -> [w746 w759 _ _]
    tunnel: w114 -> [w745 _ _ _]
    tunnel: w113 -> [w744 _ _ _]
    tunnel: w112 -> [w743 w758 w769 w776]
    tunnel: [w742 w757 w768 _] -> w21
    tunnel: [w741 w756 w767 _] -> w20
    tunnel: [w740 w755 _ _] -> w19
    tunnel: [w739 w754 _ _] -> w18
    tunnel: [w738 _ _ _] -> w17
    tunnel: [w737 _ _ _] -> w16
    frame 4, Default {
      n173 = call-poly <vilib>:"DAQmx Trigger.vi"("task/channels in"=w753, "source"=w743, "error in"=w752) -> ("task out"=w751:refnum<k21>, "error out"=w750:errorcluster)  [unwired: 11 in]
      n174 = call-poly <vilib>:"DAQmx Trigger.vi"("task/channels in"=w748, "source"=w743, "error in"=w749) -> ("task out"=w741:refnum<k21>, "error out"=w742:errorcluster)  [unwired: 11 in]
      n175 = call-poly <vilib>:"DAQmx Trigger.vi"("task/channels in"=w747, "source"=w743, "error in"=w746) -> ("task out"=w740:refnum<k21>, "error out"=w739:errorcluster)  [unwired: 11 in]
      n176 = call-poly <vilib>:"DAQmx Trigger.vi"("task/channels in"=w744, "source"=w743, "error in"=w745) -> ("task out"=w737:refnum<k21>, "error out"=w738:errorcluster)  [unwired: 11 in]
    }
    frame 3 {
      n177 = call-poly <vilib>:"DAQmx Trigger.vi"("task/channels in"=w766, "source"=w758, "error in"=w765) -> ("task out"=w764:refnum<k21>, "error out"=w763:errorcluster)  [unwired: 11 in]
      n178 = call-poly <vilib>:"DAQmx Trigger.vi"("task/channels in"=w761, "source"=w758, "error in"=w762) -> ("task out"=w756:refnum<k21>, "error out"=w757:errorcluster)  [unwired: 11 in]
      n179 = call-poly <vilib>:"DAQmx Trigger.vi"("task/channels in"=w760, "source"=w758, "error in"=w759) -> ("task out"=w755:refnum<k21>, "error out"=w754:errorcluster)  [unwired: 11 in]
    }
    frame 2 {
      n180 = call-poly <vilib>:"DAQmx Trigger.vi"("task/channels in"=w775, "source"=w769, "error in"=w774) -> ("task out"=w773:refnum<k21>, "error out"=w772:errorcluster)  [unwired: 11 in]
      n181 = call-poly <vilib>:"DAQmx Trigger.vi"("task/channels in"=w770, "source"=w769, "error in"=w771) -> ("task out"=w767:refnum<k21>, "error out"=w768:errorcluster)  [unwired: 11 in]
    }
    frame 1 {
      n182 = call-poly <vilib>:"DAQmx Trigger.vi"("task/channels in"=w780, "source"=w776, "error in"=w779) -> ("task out"=w778:refnum<k21>, "error out"=w777:errorcluster)  [unwired: 11 in]
    }
  }
  n183 = case shown="1" w179 {
    tunnel: w133 -> [w793 w802 w807 _]
    tunnel: w132 -> [w792 w801 w806 _]
    tunnel: w131 -> [w791 w800 _ _]
    tunnel: w130 -> [w790 w799 _ _]
    tunnel: w125 -> [w789 _ _ _]
    tunnel: w124 -> [w788 _ _ _]
    tunnel: w112 -> [w787 w798 w805 _]
    tunnel: [w786 _ _ _] -> w27
    tunnel: [w785 w797 _ _] -> w26
    tunnel: [w784 w796 w804 _] -> w25
    tunnel: [w783 w795 w803 _] -> w24
    tunnel: [w782 w794 _ _] -> w23
    tunnel: [w781 _ _ _] -> w22
    frame 4, Default {
      n184 = call-poly <vilib>:"DAQmx Trigger.vi"("task/channels in"=w793, "source"=w787, "error in"=w792) -> ("task out"=w784:refnum<k21>, "error out"=w783:errorcluster)  [unwired: 11 in]
      n185 = call-poly <vilib>:"DAQmx Trigger.vi"("task/channels in"=w790, "source"=w787, "error in"=w791) -> ("task out"=w785:refnum<k21>, "error out"=w782:errorcluster)  [unwired: 11 in]
      n186 = call-poly <vilib>:"DAQmx Trigger.vi"("task/channels in"=w789, "source"=w787, "error in"=w788) -> ("task out"=w786:refnum<k21>, "error out"=w781:errorcluster)  [unwired: 11 in]
    }
    frame 3 {
      n187 = call-poly <vilib>:"DAQmx Trigger.vi"("task/channels in"=w802, "source"=w798, "error in"=w801) -> ("task out"=w796:refnum<k21>, "error out"=w795:errorcluster)  [unwired: 11 in]
      n188 = call-poly <vilib>:"DAQmx Trigger.vi"("task/channels in"=w799, "source"=w798, "error in"=w800) -> ("task out"=w797:refnum<k21>, "error out"=w794:errorcluster)  [unwired: 11 in]
    }
    frame 2 {
      n189 = call-poly <vilib>:"DAQmx Trigger.vi"("task/channels in"=w807, "source"=w805, "error in"=w806) -> ("task out"=w804:refnum<k21>, "error out"=w803:errorcluster)  [unwired: 11 in]
    }
    frame 1 {
    }
  }
  n190 = case shown="True" w7 {
    tunnel: w140 -> [w853 w949]
    tunnel: w139 -> [w852 w948]
    tunnel: [w851 w948] -> w138
    tunnel: [w850 w949] -> w137
    tunnel: [w849 w947] -> w123
    tunnel: w120 -> [w848 w941]
    tunnel: w119 -> [w847 w940]
    tunnel: [w846 w945] -> w111
    tunnel: [w845 w943] -> w110
    tunnel: [w844 w946] -> w109
    tunnel: [w843 w944] -> w108
    tunnel: [w842 w942] -> w107
    tunnel: [w841 w941] -> w106
    tunnel: [w840 w939] -> w105
    tunnel: [w839 w937] -> w104
    tunnel: [w838 w940] -> w103
    tunnel: [w837 w938] -> w102
    tunnel: [w836 w936] -> w101
    tunnel: [w835 w935] -> w100
    tunnel: [w834 w934] -> w99
    tunnel: w27 -> [w833 w943]
    tunnel: w26 -> [w832 w945]
    tunnel: w25 -> [w831 w947]
    tunnel: w24 -> [w830 w946]
    tunnel: w23 -> [w829 w944]
    tunnel: w22 -> [w828 w942]
    tunnel: w21 -> [w827 w938]
    tunnel: w20 -> [w826 w939]
    tunnel: w19 -> [w825 w937]
    tunnel: w18 -> [w824 w936]
    tunnel: w17 -> [w823 w934]
    tunnel: w16 -> [w822 w935]
    tunnel: w181 -> [w809 _]
    tunnel: w179 -> [w808 _]
    frame False {
      n191 = case shown="1" w808 {
        tunnel: [w918 w928 w933 _] -> w849
        tunnel: [w917 w927 _ _] -> w846
        tunnel: [w916 _ _ _] -> w845
        tunnel: [w915 w926 w932 _] -> w844
        tunnel: [w914 w925 _ _] -> w843
        tunnel: [w913 _ _ _] -> w842
        tunnel: w833 -> [w912 _ _ _]
        tunnel: w832 -> [w911 w924 _ _]
        tunnel: w831 -> [w910 w923 w931 _]
        tunnel: w830 -> [w909 w922 w930 _]
        tunnel: w829 -> [w908 w921 _ _]
        tunnel: w828 -> [w907 _ _ _]
        tunnel: [w906 w920 w929 _] -> w816
        tunnel: [w905 w919 _ _] -> w815
        tunnel: [w904 _ _ _] -> w814
        frame 4, Default {
          n192 = property class="DAQmx Timing"(reference=w910, error in=w909) -> (reference out=w918:refnum<k21>, error out=w915:errorcluster, "SyncPulse.SyncTime"=w906:dbl)
          n193 = property class="DAQmx Timing"(reference=w911, error in=w908) -> (reference out=w917:refnum<k21>, error out=w914:errorcluster, "SyncPulse.SyncTime"=w905:dbl)
          n194 = property class="DAQmx Timing"(reference=w912, error in=w907) -> (reference out=w916:refnum<k21>, error out=w913:errorcluster, "SyncPulse.SyncTime"=w904:dbl)
        }
        frame 3 {
          n195 = property class="DAQmx Timing"(reference=w923, error in=w922) -> (reference out=w928:refnum<k21>, error out=w926:errorcluster, "SyncPulse.SyncTime"=w920:dbl)
          n196 = property class="DAQmx Timing"(reference=w924, error in=w921) -> (reference out=w927:refnum<k21>, error out=w925:errorcluster, "SyncPulse.SyncTime"=w919:dbl)
        }
        frame 2 {
          n197 = property class="DAQmx Timing"(reference=w931, error in=w930) -> (reference out=w933:refnum<k21>, error out=w932:errorcluster, "SyncPulse.SyncTime"=w929:dbl)
        }
        frame 1 {
        }
      }
      n198 = case shown="1" w809 {
        tunnel: w848 -> [w873 w888 w898 w903]
        tunnel: w847 -> [w872 w887 w897 w902]
        tunnel: [w871 w886 w896 w901] -> w841
        tunnel: [w870 w885 w895 _] -> w840
        tunnel: [w869 w884 _ _] -> w839
        tunnel: [w868 w883 w894 w900] -> w838
        tunnel: [w867 w882 w893 _] -> w837
        tunnel: [w866 w881 _ _] -> w836
        tunnel: [w865 _ _ _] -> w835
        tunnel: [w864 _ _ _] -> w834
        tunnel: w827 -> [w863 w880 w892 _]
        tunnel: w826 -> [w862 w879 w891 _]
        tunnel: w825 -> [w861 w878 _ _]
        tunnel: w824 -> [w860 w877 _ _]
        tunnel: w823 -> [w859 _ _ _]
        tunnel: w822 -> [w858 _ _ _]
        tunnel: [w857 w876 w890 w899] -> w813
        tunnel: [w856 w875 w889 _] -> w812
        tunnel: [w855 w874 _ _] -> w811
        tunnel: [w854 _ _ _] -> w810
        frame 4, Default {
          n199 = property class="DAQmx Timing"(reference=w873, error in=w872) -> (reference out=w871:refnum<k21>, error out=w868:errorcluster, "SyncPulse.SyncTime"=w857:dbl)
          n200 = property class="DAQmx Timing"(reference=w862, error in=w863) -> (reference out=w870:refnum<k21>, error out=w867:errorcluster, "SyncPulse.SyncTime"=w856:dbl)
          n201 = property class="DAQmx Timing"(reference=w861, error in=w860) -> (reference out=w869:refnum<k21>, error out=w866:errorcluster, "SyncPulse.SyncTime"=w855:dbl)
          n202 = property class="DAQmx Timing"(reference=w858, error in=w859) -> (reference out=w865:refnum<k21>, error out=w864:errorcluster, "SyncPulse.SyncTime"=w854:dbl)
        }
        frame 3 {
          n203 = property class="DAQmx Timing"(reference=w888, error in=w887) -> (reference out=w886:refnum<k21>, error out=w883:errorcluster, "SyncPulse.SyncTime"=w876:dbl)
          n204 = property class="DAQmx Timing"(reference=w879, error in=w880) -> (reference out=w885:refnum<k21>, error out=w882:errorcluster, "SyncPulse.SyncTime"=w875:dbl)
          n205 = property class="DAQmx Timing"(reference=w878, error in=w877) -> (reference out=w884:refnum<k21>, error out=w881:errorcluster, "SyncPulse.SyncTime"=w874:dbl)
        }
        frame 2 {
          n206 = property class="DAQmx Timing"(reference=w898, error in=w897) -> (reference out=w896:refnum<k21>, error out=w894:errorcluster, "SyncPulse.SyncTime"=w890:dbl)
          n207 = property class="DAQmx Timing"(reference=w891, error in=w892) -> (reference out=w895:refnum<k21>, error out=w893:errorcluster, "SyncPulse.SyncTime"=w889:dbl)
        }
        frame 1 {
          n208 = property class="DAQmx Timing"(reference=w903, error in=w902) -> (reference out=w901:refnum<k21>, error out=w900:errorcluster, "SyncPulse.SyncTime"=w899:dbl)
        }
      }
      n209 = property class="DAQmx Timing"(reference=w853, error in=w852) -> (reference out=w819:refnum<k21>, error out=w820:errorcluster, "SyncPulse.SyncTime"=w821:dbl)
      n210 = Build Array(w821, w816, w815, w814, w813, w812, w811, w810) -> (w818:dbl[])
      n211 = Array Max & Min(array=w818) -> (max value=w817:dbl)  [unwired: 3 out]
      n212 = property class="DAQmx Timing"(reference=w819, error in=w820, "SyncPulse.MinDelayToStart"=w817) -> (reference out=w850:refnum<k21>, error out=w851:errorcluster)
    }
    frame True {
    }
  }
  n213 = Not(x=w184) -> (.not. x?=w183:bool)
  n214 = call "4461 - Create AO waveforms.vi"("error in (no error)"="error in", "sampling info"="sampling info", "reset signal"=w183, "AO"="AO") -> ("error out"=w5:errorcluster, "AO Array"=w80:waveform(dbl)[])  [unwired: 4 in, 2 out]
  n215 = call "4461 - Create Reference Waveforms.vi"("sampling info"="sampling info", "reset signal"=w183, "Lockin"="Channels: Lockin") -> ()  [unwired: 5 in, 4 out]
  n216 = Index Array(array=w80) -> (element #1=w84:waveform(dbl), element #3=w94:waveform(dbl), element #4=w93:waveform(dbl), element #5=w92:waveform(dbl), element #6=w91:waveform(dbl), element #7=w90:waveform(dbl), element #8=w89:waveform(dbl))  [unwired: 8 in, 1 out]
  n217 = Build Array(w84) -> (w88:waveform(dbl)[])
  n218 = Build Array(w94, w93) -> (w87:waveform(dbl)[])
  n219 = Build Array(w92, w91) -> (w86:waveform(dbl)[])
  n220 = Build Array(w90, w89) -> (w85:waveform(dbl)[])
  n221 = flat-sequence {
    tunnel: w138 -> [w975]
    tunnel: w137 -> [w976]
    tunnel: [w976] -> w178
    tunnel: [w975] -> w177
    tunnel: [w974] -> w176
    tunnel: w123 -> [w974]
    tunnel: [w973] -> w175
    tunnel: w111 -> [w973]
    tunnel: [w972] -> w174
    tunnel: w110 -> [w972]
    tunnel: [w971] -> w173
    tunnel: w109 -> [w971]
    tunnel: [w970] -> w172
    tunnel: w108 -> [w970]
    tunnel: [w969] -> w171
    tunnel: w107 -> [w969]
    tunnel: [w968] -> w170
    tunnel: w106 -> [w968]
    tunnel: [w956] -> w169
    tunnel: w105 -> [w957]
    tunnel: [w960] -> w168
    tunnel: w104 -> [w959]
    tunnel: [w967] -> w167
    tunnel: w103 -> [w967]
    tunnel: w102 -> [w958]
    tunnel: [w961] -> w166
    tunnel: w101 -> [w962]
    tunnel: [w963] -> w165
    tunnel: w100 -> [w966]
    tunnel: [w964] -> w164
    tunnel: w99 -> [w965]
    tunnel: [w955] -> w163
    tunnel: [w954] -> w162
    tunnel: w88 -> [w954]
    tunnel: w87 -> [w953]
    tunnel: w86 -> [w952]
    tunnel: w85 -> [w951]
    tunnel: w181 -> [w950]
    tunnel: [w1025] -> w161
    tunnel: [w1024] -> w160
    tunnel: w178 -> [w1025]
    tunnel: w177 -> [w1024]
    tunnel: [w1023] -> w159
    tunnel: w176 -> [w1023]
    tunnel: [w1022] -> w158
    tunnel: w175 -> [w1022]
    tunnel: [w1021] -> w157
    tunnel: w174 -> [w1021]
    tunnel: [w1020] -> w156
    tunnel: w173 -> [w1020]
    tunnel: [w1019] -> w155
    tunnel: w172 -> [w1019]
    tunnel: [w1018] -> w154
    tunnel: w171 -> [w1018]
    tunnel: [w1010] -> w153
    tunnel: w170 -> [w1011]
    tunnel: [w1017] -> w152
    tunnel: w169 -> [w1017]
    tunnel: [w1016] -> w151
    tunnel: w168 -> [w1016]
    tunnel: [w1009] -> w150
    tunnel: w167 -> [w1008]
    tunnel: [w1015] -> w149
    tunnel: [w1014] -> w148
    tunnel: w166 -> [w1014]
    tunnel: [w1013] -> w147
    tunnel: w165 -> [w1013]
    tunnel: [w1012] -> w146
    tunnel: w164 -> [w1012]
    tunnel: w163 -> [w1015]
    tunnel: w162 -> [w1007]
    tunnel: [w1057] -> w144
    tunnel: [w1056] -> w143
    tunnel: w161 -> [w1057]
    tunnel: w160 -> [w1056]
    tunnel: w159 -> [w1055]
    tunnel: w158 -> [w1054]
    tunnel: w157 -> [w1053]
    tunnel: w156 -> [w1052]
    tunnel: w155 -> [w1051]
    tunnel: w154 -> [w1050]
    tunnel: w153 -> [w1049]
    tunnel: w152 -> [w1048]
    tunnel: w151 -> [w1047]
    tunnel: w150 -> [w1046]
    tunnel: w149 -> [w1045]
    tunnel: w148 -> [w1044]
    tunnel: w147 -> [w1043]
    tunnel: w146 -> [w1042]
    tunnel: [w1041] -> w52
    tunnel: [w1040] -> w51
    tunnel: [w1039] -> w50
    tunnel: [w1038] -> w98
    tunnel: [w1037] -> w97
    tunnel: [w1036] -> w96
    tunnel: [w1035] -> w35
    tunnel: [w1034] -> w47
    tunnel: [w1033] -> w48
    tunnel: [w1032] -> w49
    tunnel: [w1031] -> w39
    tunnel: [w1030] -> w83
    tunnel: [w1029] -> w82
    tunnel: [w1028] -> w81
    tunnel: w179 -> [w1027]
    tunnel: w181 -> [w1026]
    frame #0 {
      n222 = case shown="2" w950 {
        tunnel: w966 -> [w991 _ _ _]
        tunnel: w965 -> [w990 _ _ _]
        tunnel: [w989 _ _ _] -> w964
        tunnel: [w988 _ _ _] -> w963
        tunnel: w962 -> [w987 w1001 _ _]
        tunnel: [w986 w1000 _ _] -> w961
        tunnel: [w985 w999 _ _] -> w960
        tunnel: w959 -> [w984 w998 _ _]
        tunnel: w958 -> [w983 w997 w1006 _]
        tunnel: w957 -> [w982 w996 w1005 _]
        tunnel: [w981 w995 w1004 _] -> w956
        tunnel: [w980 w994 w1003 _] -> w955
        tunnel: w953 -> [w979 w993 w1002 _]
        tunnel: w952 -> [w978 w992 _ _]
        tunnel: w951 -> [w977 _ _ _]
        frame 4, Default {
          n223 = call-poly <vilib>:"DAQmx Write.vi"("task/channels in"=w984, "data"=w978, "error in"=w987) -> ("task out"=w985:refnum<k21>, "error out"=w986:errorcluster)  [unwired: 10 in, 1 out]
          n224 = call-poly <vilib>:"DAQmx Write.vi"("task/channels in"=w991, "data"=w977, "error in"=w990) -> ("task out"=w988:refnum<k21>, "error out"=w989:errorcluster)  [unwired: 10 in, 1 out]
          n225 = call-poly <vilib>:"DAQmx Write.vi"("task/channels in"=w982, "data"=w979, "error in"=w983) -> ("task out"=w981:refnum<k21>, "error out"=w980:errorcluster)  [unwired: 10 in, 1 out]
        }
        frame 3 {
          n226 = call-poly <vilib>:"DAQmx Write.vi"("task/channels in"=w998, "data"=w992, "error in"=w1001) -> ("task out"=w999:refnum<k21>, "error out"=w1000:errorcluster)  [unwired: 10 in, 1 out]
          n227 = call-poly <vilib>:"DAQmx Write.vi"("task/channels in"=w996, "data"=w993, "error in"=w997) -> ("task out"=w995:refnum<k21>, "error out"=w994:errorcluster)  [unwired: 10 in, 1 out]
        }
        frame 2 {
          n228 = call-poly <vilib>:"DAQmx Write.vi"("task/channels in"=w1005, "data"=w1002, "error in"=w1006) -> ("task out"=w1004:refnum<k21>, "error out"=w1003:errorcluster)  [unwired: 10 in, 1 out]
        }
        frame 1 {
        }
      }
    }
    frame #1 {
      n229 = call-poly <vilib>:"DAQmx Write.vi"("task/channels in"=w1011, "data"=w1007, "error in"=w1008) -> ("task out"=w1010:refnum<k21>, "error out"=w1009:errorcluster)  [unwired: 10 in, 1 out]
    }
    frame #2 {
      n230 = case shown="3" w1027 {
        tunnel: w1055 -> [w1109 w1117 w1121 _]
        tunnel: w1054 -> [w1108 w1116 _ _]
        tunnel: w1053 -> [w1107 _ _ _]
        tunnel: w1052 -> [w1106 w1115 w1120 _]
        tunnel: w1051 -> [w1105 w1114 _ _]
        tunnel: w1050 -> [w1104 _ _ _]
        tunnel: [w1103 w1113 w1119 _] -> w1041
        tunnel: [w1102 w1112 _ _] -> w1040
        tunnel: [w1101 _ _ _] -> w1039
        tunnel: [w1100 w1111 w1118 _] -> w1034
        tunnel: [w1099 w1110 _ _] -> w1033
        tunnel: [w1098 _ _ _] -> w1032
        frame 4, Default {
          n231 = call <vilib>:"DAQmx Start Task.vi"("task/channels in"=w1109, "error in"=w1106) -> ("task out"=w1103:refnum<k21>, "error out"=w1100:errorcluster)  [unwired: 12 in]
          n232 = call <vilib>:"DAQmx Start Task.vi"("task/channels in"=w1108, "error in"=w1105) -> ("task out"=w1102:refnum<k21>, "error out"=w1099:errorcluster)  [unwired: 12 in]
          n233 = call <vilib>:"DAQmx Start Task.vi"("task/channels in"=w1107, "error in"=w1104) -> ("task out"=w1101:refnum<k21>, "error out"=w1098:errorcluster)  [unwired: 12 in]
        }
        frame 3 {
          n234 = call <vilib>:"DAQmx Start Task.vi"("task/channels in"=w1117, "error in"=w1115) -> ("task out"=w1113:refnum<k21>, "error out"=w1111:errorcluster)  [unwired: 12 in]
          n235 = call <vilib>:"DAQmx Start Task.vi"("task/channels in"=w1116, "error in"=w1114) -> ("task out"=w1112:refnum<k21>, "error out"=w1110:errorcluster)  [unwired: 12 in]
        }
        frame 2 {
          n236 = call <vilib>:"DAQmx Start Task.vi"("task/channels in"=w1121, "error in"=w1120) -> ("task out"=w1119:refnum<k21>, "error out"=w1118:errorcluster)  [unwired: 12 in]
        }
        frame 1 {
        }
      }
      n237 = case shown="1" w1026 {
        tunnel: w1049 -> [w1073 w1085 w1093 w1097]
        tunnel: w1048 -> [w1072 w1084 w1092 _]
        tunnel: w1047 -> [w1071 w1083 _ _]
        tunnel: w1046 -> [w1070 w1082 w1091 w1096]
        tunnel: w1045 -> [w1069 w1081 w1090 _]
        tunnel: w1044 -> [w1068 w1080 _ _]
        tunnel: w1043 -> [w1067 _ _ _]
        tunnel: w1042 -> [w1066 _ _ _]
        tunnel: [w1065 w1079 w1089 w1095] -> w1038
        tunnel: [w1064 w1078 w1088 _] -> w1037
        tunnel: [w1063 w1077 _ _] -> w1036
        tunnel: [w1062 _ _ _] -> w1035
        tunnel: [w1061 w1076 w1087 w1094] -> w1031
        tunnel: [w1060 w1075 w1086 _] -> w1030
        tunnel: [w1059 w1074 _ _] -> w1029
        tunnel: [w1058 _ _ _] -> w1028
        frame 4, Default {
          n238 = call <vilib>:"DAQmx Start Task.vi"("task/channels in"=w1073, "error in"=w1070) -> ("task out"=w1065:refnum<k21>, "error out"=w1061:errorcluster)  [unwired: 12 in]
          n239 = call <vilib>:"DAQmx Start Task.vi"("task/channels in"=w1072, "error in"=w1069) -> ("task out"=w1064:refnum<k21>, "error out"=w1060:errorcluster)  [unwired: 12 in]
          n240 = call <vilib>:"DAQmx Start Task.vi"("task/channels in"=w1071, "error in"=w1068) -> ("task out"=w1063:refnum<k21>, "error out"=w1059:errorcluster)  [unwired: 12 in]
          n241 = call <vilib>:"DAQmx Start Task.vi"("task/channels in"=w1067, "error in"=w1066) -> ("task out"=w1062:refnum<k21>, "error out"=w1058:errorcluster)  [unwired: 12 in]
        }
        frame 3 {
          n242 = call <vilib>:"DAQmx Start Task.vi"("task/channels in"=w1085, "error in"=w1082) -> ("task out"=w1079:refnum<k21>, "error out"=w1076:errorcluster)  [unwired: 12 in]
          n243 = call <vilib>:"DAQmx Start Task.vi"("task/channels in"=w1084, "error in"=w1081) -> ("task out"=w1078:refnum<k21>, "error out"=w1075:errorcluster)  [unwired: 12 in]
          n244 = call <vilib>:"DAQmx Start Task.vi"("task/channels in"=w1083, "error in"=w1080) -> ("task out"=w1077:refnum<k21>, "error out"=w1074:errorcluster)  [unwired: 12 in]
        }
        frame 2 {
          n245 = call <vilib>:"DAQmx Start Task.vi"("task/channels in"=w1093, "error in"=w1091) -> ("task out"=w1089:refnum<k21>, "error out"=w1087:errorcluster)  [unwired: 12 in]
          n246 = call <vilib>:"DAQmx Start Task.vi"("task/channels in"=w1092, "error in"=w1090) -> ("task out"=w1088:refnum<k21>, "error out"=w1086:errorcluster)  [unwired: 12 in]
        }
        frame 1 {
          n247 = call <vilib>:"DAQmx Start Task.vi"("task/channels in"=w1097, "error in"=w1096) -> ("task out"=w1095:refnum<k21>, "error out"=w1094:errorcluster)  [unwired: 12 in]
        }
      }
    }
  }
  n248 = call <vilib>:"DAQmx Start Task.vi"("task/channels in"=w144, "error in"=w143) -> ("task out"=w53:refnum<k21>, "error out"=w28:errorcluster)  [unwired: 12 in]
  n249 = while {
    tunnel: w53 -> [w1140]
    tunnel: w28 -> [w1139]
    tunnel: [w1123] -> w40
    tunnel: [w1138] -> w54
    tunnel: w52 -> [w1137]
    tunnel: w51 -> [w1135]
    tunnel: w50 -> [w1136]
    tunnel: w49 -> [w1134]
    tunnel: w48 -> [w1133]
    tunnel: w47 -> [w1132]
    tunnel: w180 -> [w1131]
    tunnel: [w1130] -> w46
    tunnel: [w1124] -> w45
    tunnel: [w1129] -> w44
    tunnel: [w1126] -> w43
    tunnel: [w1128] -> w42
    tunnel: [w1127] -> w41
    tunnel: w179 -> [w1122]
    stop <- w1125 stop-if-true
    n250 = case shown="1" w1122 {
      tunnel: w1140 -> [w1167 w1188 w1203 w1212]
      tunnel: w1139 -> [w1166 w1187 w1202 w1211]
      tunnel: [w1165 w1186 w1201 w1210] -> w1138
      tunnel: w1137 -> [w1164 w1185 w1200 _]
      tunnel: w1136 -> [w1163 _ _ _]
      tunnel: w1135 -> [w1162 w1184 _ _]
      tunnel: w1134 -> [w1161 _ _ _]
      tunnel: w1133 -> [w1160 w1183 _ _]
      tunnel: w1132 -> [w1159 w1182 w1199 _]
      tunnel: w1131 -> [w1158 w1181 w1198 w1209]
      tunnel: [w1153 w1177 w1195 _] -> w1130
      tunnel: [w1152 w1176 _ _] -> w1129
      tunnel: [w1151 _ _ _] -> w1128
      tunnel: [w1150 _ _ _] -> w1127
      tunnel: [w1149 w1175 _ _] -> w1126
      tunnel: [w1148 w1174 w1194 w1207] -> w1125
      tunnel: [w1147 w1173 w1193 _] -> w1124
      tunnel: [w1146 w1172 w1192 w1206] -> w1123
      frame 4, Default {
        n251 = property class="DAQmx Read"(reference=w1167, error in=w1166) -> (reference out=w1165:refnum<k21>, error out=w1146:errorcluster, "AvailSampPerChan"=w1144:u32)
        n252 = property class="DAQmx Read"(reference=w1164, error in=w1159) -> (reference out=w1153:refnum<k21>, error out=w1147:errorcluster, "AvailSampPerChan"=w1143:u32)
        n253 = property class="DAQmx Read"(reference=w1162, error in=w1160) -> (reference out=w1152:refnum<k21>, error out=w1149:errorcluster, "AvailSampPerChan"=w1142:u32)
        n254 = property class="DAQmx Read"(reference=w1163, error in=w1161) -> (reference out=w1151:refnum<k21>, error out=w1150:errorcluster, "AvailSampPerChan"=w1141:u32)
        n255 = Greater Or Equal?(x=w1144, y=w1158) -> (x >= y?=w1157:bool)
        n256 = Greater Or Equal?(x=w1143, y=w1158) -> (x >= y?=w1156:bool)
        n257 = Greater Or Equal?(x=w1142, y=w1158) -> (x >= y?=w1155:bool)
        n258 = Greater Or Equal?(x=w1141, y=w1158) -> (x >= y?=w1154:bool)
        n259 = Compound Arithmetic op=AND(w1157, w1156, w1155, w1154) -> (w1145:bool)
        n260 = Compound Arithmetic op=OR(w1146, w1147, w1149, w1150, w1145) -> (w1148:bool)
      }
      frame 3 {
        n261 = property class="DAQmx Read"(reference=w1188, error in=w1187) -> (reference out=w1186:refnum<k21>, error out=w1172:errorcluster, "AvailSampPerChan"=w1170:u32)
        n262 = property class="DAQmx Read"(reference=w1185, error in=w1182) -> (reference out=w1177:refnum<k21>, error out=w1173:errorcluster, "AvailSampPerChan"=w1169:u32)
        n263 = property class="DAQmx Read"(reference=w1184, error in=w1183) -> (reference out=w1176:refnum<k21>, error out=w1175:errorcluster, "AvailSampPerChan"=w1168:u32)
        n264 = Greater Or Equal?(x=w1170, y=w1181) -> (x >= y?=w1180:bool)
        n265 = Greater Or Equal?(x=w1169, y=w1181) -> (x >= y?=w1179:bool)
        n266 = Greater Or Equal?(x=w1168, y=w1181) -> (x >= y?=w1178:bool)
        n267 = Compound Arithmetic op=AND(w1180, w1179, w1178) -> (w1171:bool)
        n268 = Compound Arithmetic op=OR(w1172, w1173, w1175, w1171) -> (w1174:bool)
      }
      frame 2 {
        n269 = property class="DAQmx Read"(reference=w1203, error in=w1202) -> (reference out=w1201:refnum<k21>, error out=w1192:errorcluster, "AvailSampPerChan"=w1190:u32)
        n270 = property class="DAQmx Read"(reference=w1200, error in=w1199) -> (reference out=w1195:refnum<k21>, error out=w1193:errorcluster, "AvailSampPerChan"=w1189:u32)
        n271 = Greater Or Equal?(x=w1190, y=w1198) -> (x >= y?=w1197:bool)
        n272 = Greater Or Equal?(x=w1189, y=w1198) -> (x >= y?=w1196:bool)
        n273 = Compound Arithmetic op=AND(w1197, w1196) -> (w1191:bool)
        n274 = Compound Arithmetic op=OR(w1192, w1193, w1191) -> (w1194:bool)
      }
      frame 1 {
        n275 = property class="DAQmx Read"(reference=w1212, error in=w1211) -> (reference out=w1210:refnum<k21>, error out=w1206:errorcluster, "AvailSampPerChan"=w1204:u32)
        n276 = Greater Or Equal?(x=w1204, y=w1209) -> (x >= y?=w1208:bool)
        n277 = Compound Arithmetic op=AND(w1208) -> (w1205:bool)
        n278 = Compound Arithmetic op=OR(w1206, w1205) -> (w1207:bool)
      }
    }
  }
  n279 = case shown="3" w179 {
    tunnel: [w1231 w1246 w1257 w1264] -> w205
    tunnel: w54 -> [w1230 w1245 w1256 w1263]
    tunnel: w46 -> [w1229 w1244 w1255 _]
    tunnel: w45 -> [w1228 w1243 w1254 _]
    tunnel: w44 -> [w1227 w1242 _ _]
    tunnel: w43 -> [w1226 w1241 _ _]
    tunnel: w42 -> [w1225 _ _ _]
    tunnel: w41 -> [w1224 _ _ _]
    tunnel: w40 -> [w1223 w1240 w1253 w1262]
    tunnel: w180 -> [w1215 w1234 w1249 w1260]
    tunnel: [w1213 w1232 w1247 w1258] -> w6
    frame 4, Default {
      n280 = call-poly <vilib>:"DAQmx Read.vi"("task/channels in"=w1230, "number of samples per channel"=w1215, "error in"=w1223) -> ("task out"=w1222:refnum<k21>, "error out"=w1214:errorcluster)  [unwired: 10 in, 1 out]
      n281 = call-poly <vilib>:"DAQmx Read.vi"("task/channels in"=w1229, "number of samples per channel"=w1215, "error in"=w1228) -> ("task out"=w1221:refnum<k21>, "error out"=w1220:errorcluster)  [unwired: 10 in, 1 out]
      n282 = call-poly <vilib>:"DAQmx Read.vi"("task/channels in"=w1227, "number of samples per channel"=w1215, "error in"=w1226) -> ("task out"=w1216:refnum<k21>, "error out"=w1219:errorcluster)  [unwired: 10 in, 1 out]
      n283 = call-poly <vilib>:"DAQmx Read.vi"("task/channels in"=w1225, "number of samples per channel"=w1215, "error in"=w1224) -> ("task out"=w1217:refnum<k21>, "error out"=w1218:errorcluster)  [unwired: 10 in, 1 out]
      n284 = Build Array(w1222, w1221, w1216, w1217) -> (w1231:refnum<k21>[])
      n285 = Merge Errors(w1214, w1220, w1219, w1218) -> (w1213:errorcluster)
    }
    frame 3 {
      n286 = call-poly <vilib>:"DAQmx Read.vi"("task/channels in"=w1245, "number of samples per channel"=w1234, "error in"=w1240) -> ("task out"=w1239:refnum<k21>, "error out"=w1233:errorcluster)  [unwired: 10 in, 1 out]
      n287 = call-poly <vilib>:"DAQmx Read.vi"("task/channels in"=w1244, "number of samples per channel"=w1234, "error in"=w1243) -> ("task out"=w1238:refnum<k21>, "error out"=w1237:errorcluster)  [unwired: 10 in, 1 out]
      n288 = call-poly <vilib>:"DAQmx Read.vi"("task/channels in"=w1242, "number of samples per channel"=w1234, "error in"=w1241) -> ("task out"=w1235:refnum<k21>, "error out"=w1236:errorcluster)  [unwired: 10 in, 1 out]
      n289 = Build Array(w1239, w1238, w1235) -> (w1246:refnum<k21>[])
      n290 = Merge Errors(w1233, w1237, w1236) -> (w1232:errorcluster)
    }
    frame 2 {
      n291 = call-poly <vilib>:"DAQmx Read.vi"("task/channels in"=w1256, "number of samples per channel"=w1249, "error in"=w1253) -> ("task out"=w1252:refnum<k21>, "error out"=w1248:errorcluster)  [unwired: 10 in, 1 out]
      n292 = call-poly <vilib>:"DAQmx Read.vi"("task/channels in"=w1255, "number of samples per channel"=w1249, "error in"=w1254) -> ("task out"=w1251:refnum<k21>, "error out"=w1250:errorcluster)  [unwired: 10 in, 1 out]
      n293 = Build Array(w1252, w1251) -> (w1257:refnum<k21>[])
      n294 = Merge Errors(w1248, w1250) -> (w1247:errorcluster)
    }
    frame 1 {
      n295 = call-poly <vilib>:"DAQmx Read.vi"("task/channels in"=w1263, "number of samples per channel"=w1260, "error in"=w1262) -> ("task out"=w1261:refnum<k21>, "error out"=w1259:errorcluster)  [unwired: 10 in, 1 out]
      n296 = Build Array(w1261) -> (w1264:refnum<k21>[])
      n297 = Merge Errors(w1259) -> (w1258:errorcluster)
    }
  }
  "AI task" <- w205
  n298 = case shown="4, Default" w181 {
    tunnel: w98 -> [w1274 w1282 w1288 w1292]
    tunnel: w97 -> [w1273 w1281 w1287 _]
    tunnel: w96 -> [w1272 w1280 _ _]
    tunnel: [w1271 w1279 w1286 w1291] -> w204
    tunnel: w83 -> [w1270 w1278 w1285 _]
    tunnel: w82 -> [w1269 w1277 _ _]
    tunnel: w81 -> [w1268 _ _ _]
    tunnel: w39 -> [w1267 w1276 w1284 w1290]
    tunnel: [w1266 w1275 w1283 w1289] -> w36
    tunnel: w35 -> [w1265 _ _ _]
    frame 4, Default {
      n299 = Build Array(w1274, w1273, w1272, w1265) -> (w1271:refnum<k21>[])
      n300 = Merge Errors(w1267, w1270, w1269, w1268) -> (w1266:errorcluster)
    }
    frame 3 {
      n301 = Build Array(w1282, w1281, w1280) -> (w1279:refnum<k21>[])
      n302 = Merge Errors(w1276, w1278, w1277) -> (w1275:errorcluster)
    }
    frame 2 {
      n303 = Build Array(w1288, w1287) -> (w1286:refnum<k21>[])
      n304 = Merge Errors(w1284, w1285) -> (w1283:errorcluster)
    }
    frame 1 {
      n305 = Build Array(w1292) -> (w1291:refnum<k21>[])
      n306 = Merge Errors(w1290) -> (w1289:errorcluster)
    }
  }
  "AO Task" <- w204
  n307 = Merge Errors(w6, w36, w5) -> (→"error out":errorcluster)
